vi "COD内部交互全局.vi"() -> ()   [LabVIEW 2016, in "斯坦道CODMn.lvlib"]
panel:
  out "第一次测试时间":timestamp
  out "温度波形时间":timestamp
  out "时间-温度":u16[](array[numeric]) caption="数组"
  out "时间温度曲线":u16[](graph)
  in  "基本量程存储数据用":enum16{"L", "H", "AUTO"}(ring)
  out "报警点位":bool[](array[boolean])
  out "校准内容显示":string
  out "启用的浓度数组":dbl[](array[numeric])
  out "ORP显示":dbl
  out "波形时间":timestamp
  out "滴定数-ORP值":u16[](array[numeric]) caption="数组"
  out "ORP滴定曲线":u16[](graph)
  out "当前校准":i32
  in  "泵滴定数5":dbl
  in  "泵滴定数4":dbl
  in  "泵滴定数3":dbl
  in  "泵滴定数2":dbl
  in  "泵滴定数1":dbl
  out "实时温度":dbl
  out "高锰酸钾":dbl
  out "断电排液标记":bool
  out "报警簇":T1
  out "高锰酸钾报警":bool
  out "待机":bool
  in  "量程切换次数":u8
  out "测量模式数字":i32
  out "切换量程连续测两次":bool
  out "配置文件ini":string="data\\Set.ini"
  out "序列号:":string
  out "读取浮台参数显示":bool
  out "读取浮台参数":u16[](array[numeric])
  out "读取公式":u16[](array[numeric])
  out "读取参数":u16[](array[numeric])
  out "数据存储":u16[](array[numeric])
  out "温度":bool[](array[boolean])
  out "M输出点":bool[](array[boolean])
  out "ORP、时间":u16[](array[numeric])
  out "测量状态":u16[](array[numeric])
  out "读取公式显示":bool
  out "读取参数显示":bool
  out "读取写入data":bool
  in  "基本量程实时读取":enum16{"L", "H", "AUTO"}(ring)
  out "温度存储数据用":dbl
  out "故障标记":bool
  out "数据存储时间戳":timestamp format="%<%Y/%m/%d %H:%M:%S>T"
  out "通讯状态":bool
  out "data":T2
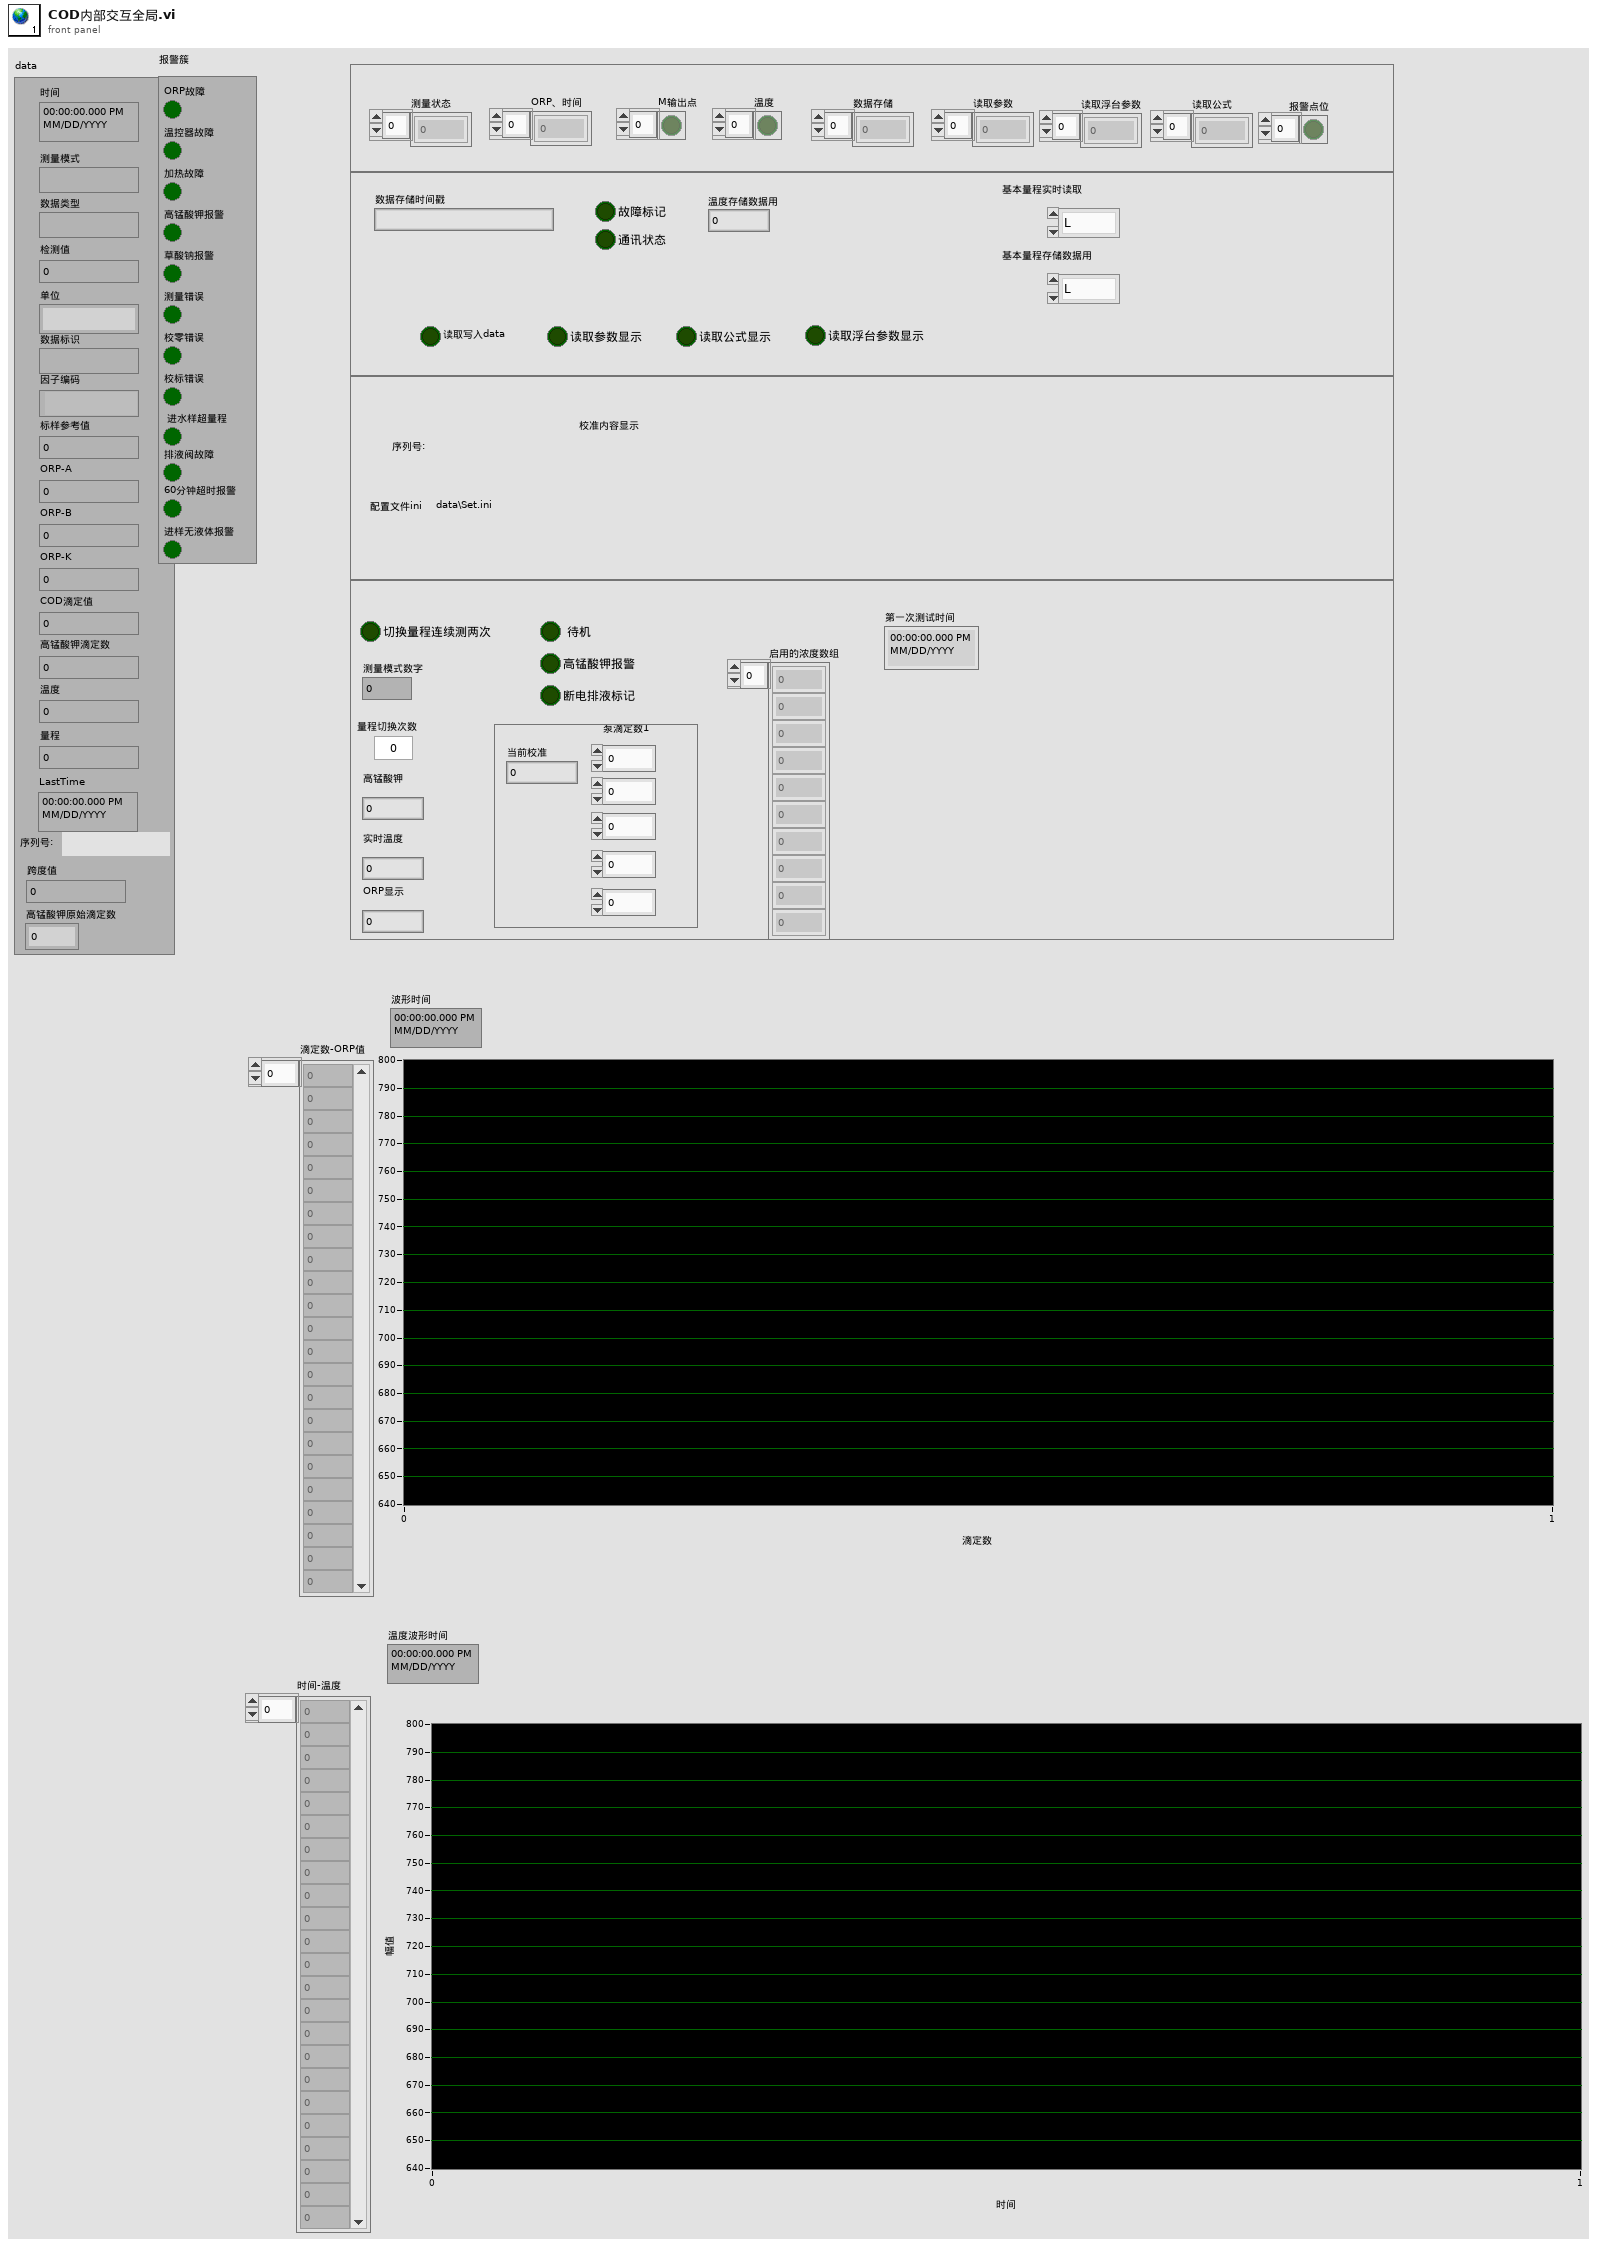
[diagram p1: front panel]
types:
  T1 = cluster{"ORP故障":bool, "温控器故障":bool, "加热故障":bool, "高锰酸钾报警":bool, "草酸钠报警":bool, "测量错误":bool, "校零错误":bool, "校标错误":bool, " 进水样超量程":bool, "排液阀故障":bool, "60分钟超时报警":bool, "进样无液体报警":bool}
  T2 = cluster{"时间":timestamp, "测量模式":string, "数据类型":string, "检测值":sgl, "单位":string, "数据标识":string, "因子编码":string, "标样参考值":sgl, "ORP-A":sgl, "ORP-B":sgl, "ORP-K":sgl, "COD滴定值":sgl, "高锰酸钾滴定数":sgl, "温度":sgl, "量程":sgl, "LastTime":timestamp, "序列号:":string, "跨度值":sgl, "高锰酸钾原始滴定数":sgl}
diagram:
